vi "Enlong Output Signal.vi"(1 "Trigger In":bool) -> (0 "Trigger Out":bool)   [LabVIEW 2014]
panel:
  # "Copyright 2014 Vidrio Technologies\nScanImage 5 software is licensed under the Apache License, Version 2.0 (the \"License\"); you may not use any files contained\nwithin the ScanImage 5 release except in compliance with the License. You may obtain a copy of the License at\n http://www.apache.org/licenses/LICENSE-2.0\nUnless required by applicable law or agreed to in writing, software distributed under the License is distributed on an\n\"AS IS\" BASIS, WITHOUT WARRANTIES OR CONDITIONS OF ANY KIND, either express or implied. See the License for the\n specific language governing permissions and limitations under the License."
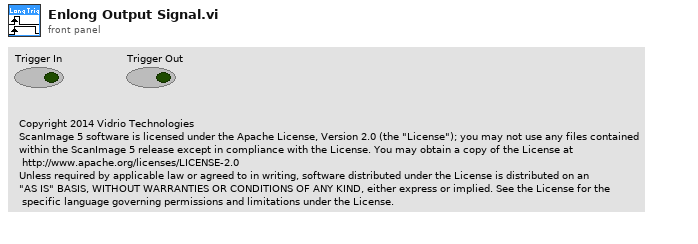
[diagram p1: front panel]
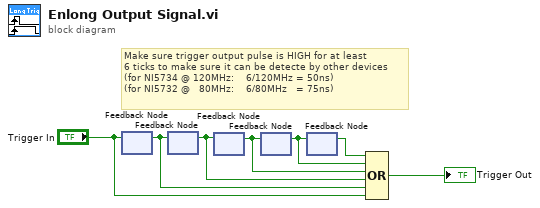
[diagram p0: block diagram]
diagram:
  # "Make sure trigger output pulse is HIGH for at least\n6 ticks to make sure it can be detecte by other devices\n(for NI5734 @ 120MHz:    6/120MHz = 50ns)\n(for NI5732 @   80MHz:    6/80MHz   = 75ns)"
  n1 = feedback #1() -> (w5:bool)  [unwired: 1 in]
  n2 = feedback-in #1("Trigger In") -> ()
  n3 = feedback #2() -> (w4:bool)  [unwired: 1 in]
  n4 = feedback-in #2(w5) -> ()
  n5 = feedback #3() -> (w3:bool)  [unwired: 1 in]
  n6 = feedback-in #3(w4) -> ()
  n7 = feedback #4() -> (w2:bool)  [unwired: 1 in]
  n8 = feedback-in #4(w3) -> ()
  n9 = feedback #5() -> (w1:bool)  [unwired: 1 in]
  n10 = feedback-in #5(w2) -> ()
  n11 = Compound Arithmetic op=OR(w1, w2, w3, w4, w5, "Trigger In") -> (→"Trigger Out":bool)
